vi "Event_Counter.vi"(1 "Counts in":u32, 2 "input":bool) -> (0 "Counts out":u32)   [LabVIEW 2014]
panel:
  # "U32 counter"
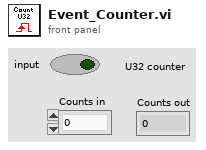
[diagram p1: front panel]
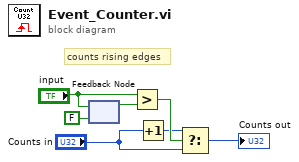
[diagram p0: block diagram]
diagram:
  # "counts rising edges"
  n1 = feedback-in #1("input") -> ()
  n2 = feedback #1(FALSE ("input")) -> (w3:bool)
  n3 = Greater?(x="input", y=w3) -> (0:w7:bool)
  n4 = Increment(x="Counts in") -> (x+1=w6:u32)
  n5 = Select(t=w6, s=w7, f="Counts in") -> (s? t:f=→"Counts out":u32)
